vi "CheckAlarms.vi"(8 "error in (no error)":errorcluster, 10 "ControlQueue":refnum<queue>, 11 "DAQmxTaksContainer_General in":refnum<class "DAQmxTaksContainer_General.lvclass">) -> (0 "error out":errorcluster, 3 "DAQmxTaksContainer_General out":refnum<class "DAQmxTaksContainer_General.lvclass">)   [LabVIEW 2015, in "DAQmxTaksContainer_General.lvclass"]
uses:
  DAQmxTaksContainer_General.lvclass
  DAQmxTaskAICurrent_General/DAQmxTaskAICurrent_General.lvclass/DAQmxTaskAICurrent_General.ctl
  DAQmxTask.lvclass
  DAQmxTaskAICurrent_General/DAQmxTaskAICurrent_General.lvclass
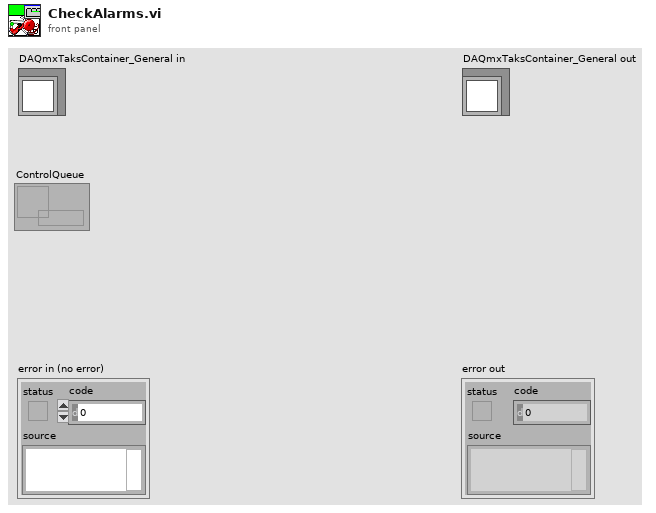
[diagram p1: front panel]
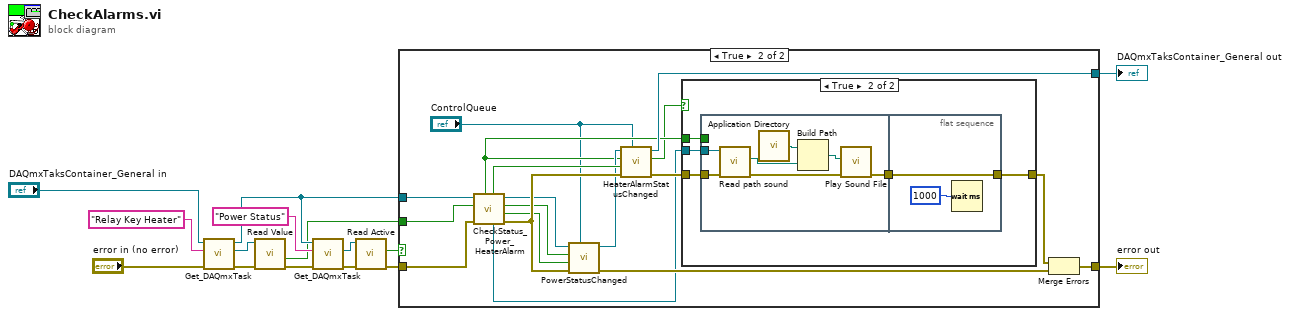
[diagram p0: block diagram]
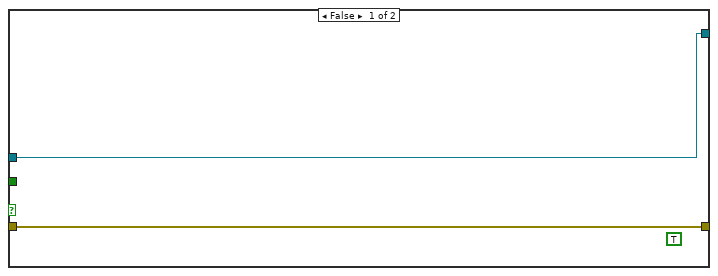
[diagram p2: hidden frame]
diagram:
  n1 = call "Get_DAQmxTask.vi"("error in (no error)"="error in (no error)", "Task name"="Relay Key Heater", "DAQmxTaksContainer_General in"="DAQmxTaksContainer_General in") -> ("error out"=w10:errorcluster, "DAQmx Task"=w9:refnum<class "DAQmxTask.lvclass">, "DAQmxTaksContainer_General out"=w8:refnum<class "DAQmxTaksContainer_General.lvclass">)  [unwired: 6 in]
  n2 = call-dynamic "Read Value.vi"("error in (no error)"=w10, "DAQmxTask en entrée"=w9) -> ("error out"=w7:errorcluster, "Data"=w6:bool)  [unwired: 6 in, 2 out]
  n3 = call "Get_DAQmxTask.vi"("error in (no error)"=w7, "Task name"="Power Status", "DAQmxTaksContainer_General in"=w8) -> ("error out"=w15:errorcluster, "DAQmx Task"=w14:refnum<class "DAQmxTask.lvclass">)  [unwired: 6 in, 1 out]
  n4 = call-dynamic "Read Active.vi"("error in (no error)"=w15, "DAQmxTask in"=w14) -> ("error out"=w13:errorcluster, "Active?"=w11:bool)  [unwired: 7 in, 1 out]
  n5 = case shown="True" w11 {
    tunnel: [w16 w31] -> w4
    tunnel: [w17 w27] -> w5
    tunnel: w13 -> [w16 w33]
    tunnel: w8 -> [w17 w34]
    tunnel: w6 -> [_ w29]
    frame False {
      (unwired) TRUE ("First Time")
    }
    frame True {
      n6 = call "CheckStatus_Power_HeaterAlarm.vi"("error in (no error)"=w33, "RelayKeyStatus"=w29, "DAQmxTaksContainer_General in"=w34) -> ("error out"=w30:errorcluster, "PowerStatus"=w28:bool, "PowerStatusChanged"=w22:bool, "DAQmxTaksContainer_General out"=w25:refnum<class "DAQmxTaksContainer_General.lvclass">, "DAQmxTaskAICurrent en sortie"=w20:refnum<class "DAQmxTaskAICurrent_General.lvclass">, "HeaterAlarmStatus"=w26:bool, "HeaterAlarmStatusChanged"=w21:bool)  [unwired: 2 in]
      n7 = call "PowerStatusChanged.vi"("ControlQueue"="ControlQueue", "error in (no error)"=w30, "PowerStatus"=w28, "PowerStatusChanged"=w22, "DAQmxTaksContainer_General in"=w25) -> ("error out"=w24:errorcluster, "DAQmxTaksContainer_General out"=w23:refnum<class "DAQmxTaksContainer_General.lvclass">)  [unwired: 5 in]
      n8 = call "HeaterAlarmStatusChanged.vi"("ControlQueue"="ControlQueue", "error in (no error)"=w30, "HeaterAlarmStatus"=w26, "HeaterAlarmStatusChanged"=w21, "DAQmxTaksContainer_General in"=w23) -> ("error out"=w35:errorcluster, "Alarm"=w19:bool, "DAQmxTaksContainer_General out"=w27:refnum<class "DAQmxTaksContainer_General.lvclass">)  [unwired: 4 in]
      n9 = case shown="True" w19 {
        tunnel: w35 -> [w36 w41]
        tunnel: [w36 w40] -> w32
        tunnel: w21 -> [_ w39]
        tunnel: w20 -> [_ w37]
        frame False {
        }
        frame True {
          n10 = flat-sequence {
            tunnel: w41 -> [w47]
            tunnel: w39 -> [_]
            tunnel: [w46] -> w38
            tunnel: w37 -> [w45]
            tunnel: [w50] -> w40
            tunnel: w38 -> [w50]
            frame #0 {
              n11 = call "Read path sound.vi"("error in (no error)"=w47, "DAQmxTaskAICurrent_General in"=w45) -> ("error out"=w48:errorcluster, "path sound"=w43:path)  [unwired: 7 in, 1 out]
              n12 = call <vilib>:"Application Directory.vi"() -> ("Application Directory"=w44:path)
              n13 = Build Path(base path=w44, name or relative path=w43) -> (appended path=w42:path)
              n14 = call <vilib>:"Play Sound File.vi"("error in (no error)"=w48, "path"=w42) -> ("error out"=w46:errorcluster)  [unwired: 8 in, 1 out]
            }
            frame #1 {
              n15 = Wait (ms)(milliseconds to wait=u32 1000 ("attente (ms)")) -> ()  [unwired: 1 out]
            }
          }
        }
      }
      n16 = Merge Errors(w32, w24) -> (w31:errorcluster)
    }
  }
  "error out" <- w4
  "DAQmxTaksContainer_General out" <- w5
